vi "RetriveUsersDB.vi"(9 "password":string, 10 "userID":string, 11 "connection information":path) -> (0 "error out":errorcluster, 2 "Array":string[][](array[string]))   [LabVIEW 2017]
uses:
  <vilib>/addons/database/Connection.llb/DB Tools Open Connec (Path).vi
  <vilib>/addons/database/_DB Variant To Data/Database Variant To Data.xnode
  <vilib>/addons/database/NI_Database_API.lvlib
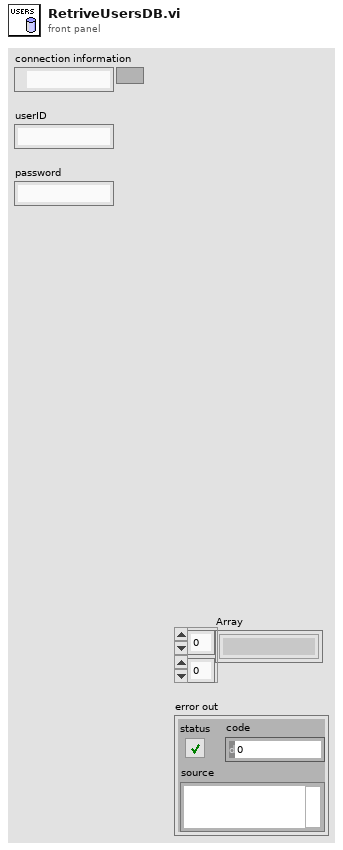
[diagram p1: front panel]
types:
  T1 = typedef "NI_Database_API.lvlib/Conn ObjectReference.ctl" = refnum<k1>
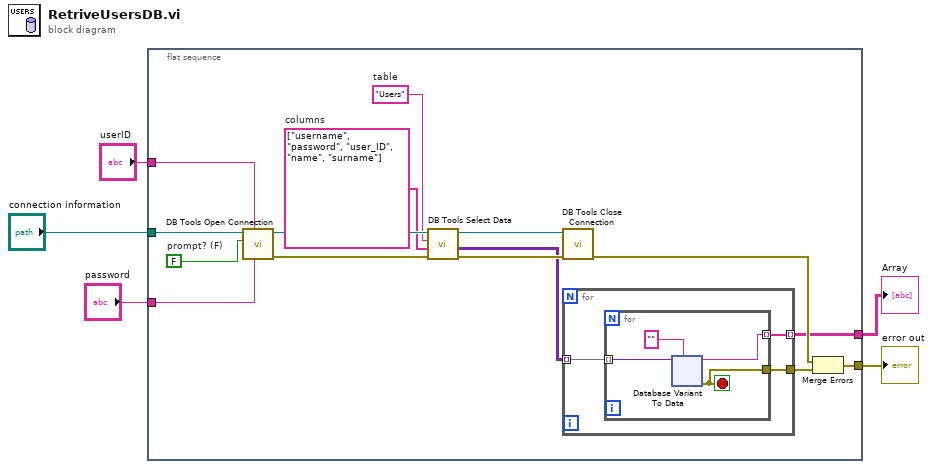
[diagram p0: block diagram]
diagram:
  n1 = flat-sequence {
    tunnel: [w10] -> w1
    tunnel: [w9] -> w2
    tunnel: "connection information" -> [w8]
    tunnel: "userID" -> [w7]
    tunnel: "password" -> [w6]
    frame #0 {
      w14 = string[] ["username", "password", "user_ID", "name", "surname"]  # columns
      w15 = "Users"  # table
      w20 = FALSE  # prompt? (F)
      n2 = call-poly <vilib>:"DB Tools Open Connection.vi"("password"=w6, "userID"=w7, "prompt? (F)"=w20, "connection information"=w8) -> ("error out"=w18:errorcluster, "connection reference"=w17:T1)  [unwired: 4 in]
      n3 = call <vilib>:"DB Tools Select Data.vi"("error in (no error)"=w18, "columns"=w14, "table"=w15, "connection reference"=w17) -> ("error out"=w16:errorcluster, "data"=w13:variant[][], "connection reference out"=w19:T1)  [unwired: 2 in]
      n4 = call <vilib>:"DB Tools Close Connection.vi"("error in (no error)"=w16, "connection reference"=w19) -> ("error out"=w12:errorcluster)  [unwired: 5 in]
      n5 = for {
        tunnel: w13 -> [w23] mode=indexing
        tunnel: [w22] -> w11
        tunnel: [w21] -> w9 mode=indexing
        n6 = for {
          tunnel: w23 -> [w27] mode=indexing
          tunnel: [w25] -> w22
          tunnel: [w24] -> w21 mode=indexing
          stop <- w25 stop-if-true
          n7 = xnode "Database Variant To Data"("database variant"=w27, "type"="") -> ("data"=w24:string, "error out"=w25:errorcluster)  [unwired: 1 in]
        }
      }
      n8 = Merge Errors(w12, w11) -> (w10:errorcluster)
    }
  }
  "Array" <- w2
  "error out" <- w1
